vi "Global Strings.vi"() -> ()   [LabVIEW 2020, in "Sequencer with Output Values.lvlib" / "Sequencer with Output Values.lvclass"]
uses:
  Sequencer with Output Values.lvclass
  Params.ctl
  Step Settings.ctl
panel:
  out "Test In Progress":bool
  in  "Total Cycles":string="Total Cycles"
  in  "Total Sequence Cycles":string="Total Sequence Cycles"
  in  "Time Left":string="Time Left"
  in  "Remaining Time in Step":string="Remaining Time in Current Step"
  in  "Step #":string="Step #"
  in  "Sequence Step":string="Sequence Step Number"
  in  "Default Initial Values":T1={"Step Values"=[], "Only Execute When Test Running"=TRUE, "Reset Sequence When Test Starts"=TRUE, "Current Sequence ID"=0, "Total Iterations"=0, "Current Step Start Timestamp"=0.0, "Number of Sequence Steps"=0, "Num of Analog Channels"=0, "Num of Digital Channels"=0, "Delay Before Starting Sequence"=0.0, "Show UI"=FALSE, "Time Remaining"=0.0, "Test Running"=FALSE, "Pause Timestamp"=0.0, "Default Analog Values"=[], "Default Digital Values"=[]}
  in  "Internal Param Message":string="Use \"Configure\" button to edit.\n\n<START>"
  in  "Internal Param":string="Internal Settings. Use \"Configure\" button to edit."
  in  "Command":string="Configure"
  in  "Delimeter":string=";"
  in  "Digital Channel Name":string="Digital Channel %d"
  in  "Analog Channel Name":string="Analog Channel %d"
  in  "Default Mode Value":string="Wait for end of step"
  in  "Mode Enum Values":string[](array[string])=["Wait for end of step", "Repeat channel values"]
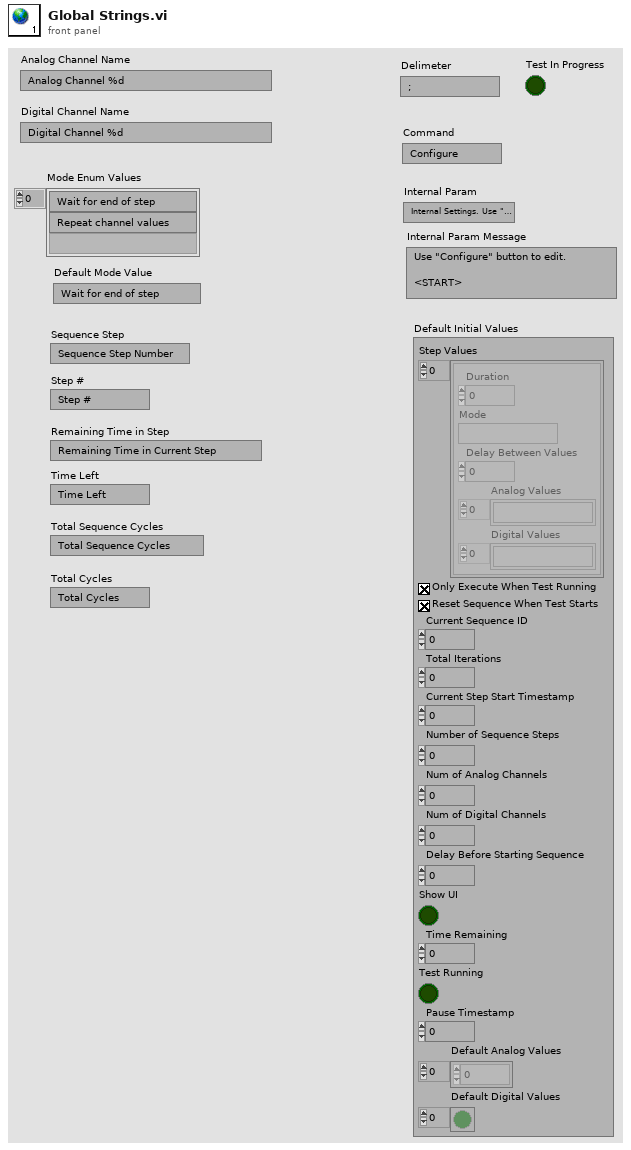
[diagram p1: front panel]
types:
  T1 = typedef "Sequencer with Output Values.lvlib/Sequencer with Output Values.lvclass/Params.ctl" = cluster{"Step Values":T2[], "Only Execute When Test Running":bool, "Reset Sequence When Test Starts":bool, "Current Sequence ID":u32, "Total Iterations":u32, "Current Step Start Timestamp":dbl, "Number of Sequence Steps":i32, "Num of Analog Channels":i32, "Num of Digital Channels":i32, "Delay Before Starting Sequence":dbl, "Show UI":bool, "Time Remaining":dbl, "Test Running":bool, "Pause Timestamp":dbl, "Default Analog Values":dbl[], "Default Digital Values":bool[]}
  T2 = typedef "Sequencer with Output Values.lvlib/Sequencer with Output Values.lvclass/Step Settings.ctl" = cluster{"Duration":dbl, "Mode":string, "Delay Between Values":dbl, "Analog Values":string[], "Digital Values":string[]}
diagram:
